vi "Test Overflow.vi"(8 "error in":errorcluster, 11 "Test Case In":refnum<class "History Tests.lvclass">) -> (0 "error out":errorcluster, 3 "Test Case Out":refnum<class "History Tests.lvclass">)   [LabVIEW 2020, in "History Tests.lvclass"]
doc: "Adds many states to the undo buffer and then performs an Undo on all of the added states."
uses:
  History Tests.lvclass
  History Tests.lvclass/History Tests.ctl
  resource/plugins/NIIconEditor/History/History/History.lvclass
panel:
  out "Undo Data":string[](array[string])
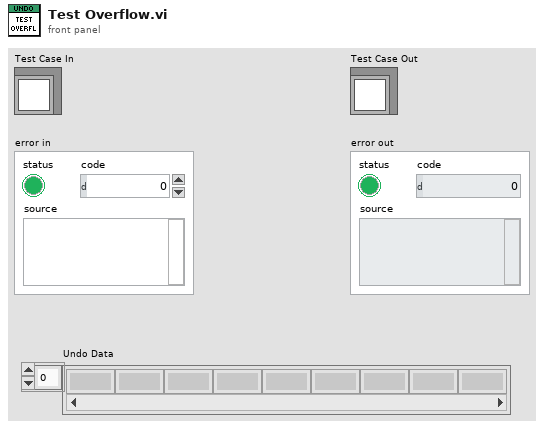
[diagram p1: front panel]
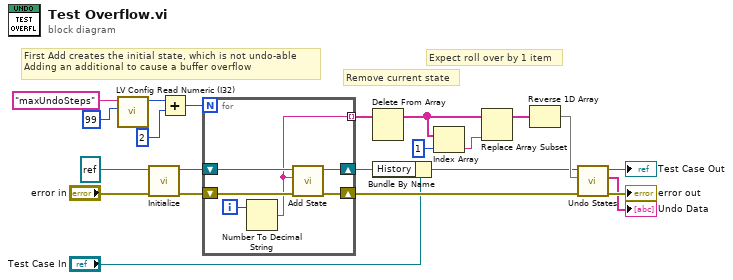
[diagram p0: block diagram]
diagram:
  # "Expect roll over by 1 item"
  # "Remove current state"
  # "First Add creates the initial state, which is not undo-able\nAdding an additional to cause a buffer overflow"
  n1 = call <resource>:"LV Config Read Numeric (I32).vi"("default value"=99, "key"="maxUndoSteps") -> ("value"=w15:i32)  [unwired: 3 in, 2 out]
  n2 = call "Initialize.vi"("error in"="error in", "menu reference"=refnum<k9> refnum) -> ("error out"=w20:errorcluster, "History"=w5:refnum<class "History.lvclass">)  [unwired: 8 in]
  n3 = Add(x=w15, y=2) -> (x+y=w14:i32)
  n4 = for {
    N: w14 -> [_]
    tunnel: [w23] -> w12 mode=indexing
    shift-right: [w24] -> w4
    shift-left: w5 -> [w25]
    shift-right: [w27] -> w19
    shift-left: w20 -> [w28]
    i -> [w26]
    n5 = Number To Decimal String(number=w26) -> (decimal integer string=w23:string)  [unwired: 1 in]
    n6 = call "Add State.vi"("error in"=w28, "State"=w23, "History in"=w25) -> ("error out"=w27:errorcluster, "History out"=w24:refnum<class "History.lvclass">)  [unwired: 7 in]
  }
  n7 = Delete From Array(array=w12) -> (array with subset deleted=w7:string[])  [unwired: 2 in, 1 out]
  n8 = Bundle By Name(cluster="Test Case In", "History"=w4) -> (w2:refnum<class "History Tests.lvclass">)
  n9 = Index Array(array=w7, index=1) -> (element=w10:string)
  n10 = Replace Array Subset(array=w7, new element=w10) -> (w9:string[])  [unwired: 1 in]
  n11 = Reverse 1D Array(array=w9) -> (reversed array=w8:string[])
  n12 = call "Undo States.vi"("error in"=w19, "Expected Undo States"=w8, "Test Case In"=w2) -> ("error out"=→"error out":errorcluster, "Actual Undo States"=→"Undo Data":string[], "Test Case Out"=→"Test Case Out":refnum<class "History Tests.lvclass">)  [unwired: 6 in]
